vi "_FPGA System Polling.vi"(4 "error in (no error)":errorcluster, 5 "Waiting (F)":bool, 6 "Connected?":bool, 7 "CurInstrState":T3) -> (1 "Running":bool, 3 "Next InstrState":T3)   [LabVIEW 2012]
uses:
  Type/_RT Instrument State.ctl
  Type/_RT Polling Settings.ctl
  Type/_LCD Line2 Msg.ctl
  Type/_LED States.ctl
  Type/_LCD Line1 Msg.ctl
  Type/_RW Status.ctl
  Type/_Pump Parameter.ctl
  _RT Global.vi
  <vilib>/Utility/error.llb/Error Cluster From Error Code.vi
  <vilib>/rvi/errors/niLvFpgaAdjustHostInterfaceError.vi
  <vilib>/rvi/interface/nirviReadWriteControl/nirviReadWriteControl.xnode
  FPGA Bitfiles/FPGA9606.lvbitx
  NiFpgaLv.dll
panel:
  in  "Polling Settings":T1[](array[typedef])=[{"ADC Ch"=119, "UserVal"=FALSE, "LowVal"=0.0, "HighVal"=89.0, "Fail Level"=50, "Err"="VG Disconnected/Broken Warning", "Line2Msg"=13, "InstrState"=enum."Ready", "Code"="004"}, {"ADC Ch"=119, "UserVal"=FALSE, "LowVal"=255.0, "HighVal"=300.0, "Fail Level"=50, "Err"="VG Disconnected/Broken Warning", "Line2Msg"=13, "InstrState"=enum."Ready", "Code"="004"}, {"ADC Ch"=119, "UserVal"=FALSE, "LowVal"=150.0, "HighVal"=254.0, "Fail Level"=50, "Err"="Overpressure Warning", "Line2Msg"=13, "InstrState"=enum."Ready", "Code"="006"}, {"ADC Ch"=64, "UserVal"=FALSE, "LowVal"=-5.0, "HighVal"=0.249, "Fail Level"=39, "Err"="Drying Gas Low", "Line2Msg"=4, "InstrState"=enum."Turbopump Ready", "Code"=""}, {"ADC Ch"=74, "UserVal"=FALSE, "LowVal"=0.36, "HighVal"=5.0, "Fail Level"=10, "Err"="Foreline Pressure Failure", "Line2Msg"=2, "InstrState"=enum."Fault", "Code"="001"}, {"ADC Ch"=25, "UserVal"=TRUE, "LowVal"=91.0, "HighVal"=200.0, "Fail Level"=35, "Err"="Q2 Board Slot 5 Overheating", "Line2Msg"=5, "InstrState"=enum."Turbopump Ready-Waiting", "Code"="008"}, {"ADC Ch"=49, "UserVal"=TRUE, "LowVal"=91.0, "HighVal"=200.0, "Fail Level"=35, "Err"="Q1 Board Slot 9 Overheating", "Line2Msg"=5, "InstrState"=enum."Turbopump Ready-Waiting", "Code"="009"}, {"ADC Ch"=57, "UserVal"=TRUE, "LowVal"=91.0, "HighVal"=200.0, "Fail Level"=35, "Err"="M1RF Board Slot 13 Overheating", "Line2Msg"=5, "InstrState"=enum."Turbopump Ready-Waiting", "Code"="010"}, {"ADC Ch"=26, "UserVal"=TRUE, "LowVal"=91.0, "HighVal"=200.0, "Fail Level"=35, "Err"="Q2 Board Slot 5 Overheating", "Line2Msg"=5, "InstrState"=enum."Turbopump Ready-Waiting", "Code"="008"}, {"ADC Ch"=50, "UserVal"=TRUE, "LowVal"=91.0, "HighVal"=200.0, "Fail Level"=35, "Err"="Q1 Board Slot 9 Overheating", "Line2Msg"=5, "InstrState"=enum."Turbopump Ready-Waiting", "Code"="009"}, {"ADC Ch"=58, "UserVal"=TRUE, "LowVal"=91.0, "HighVal"=200.0, "Fail Level"=35, "Err"="M1RF Board Slot 13 Overheating", "Line2Msg"=5, "InstrState"=enum."Turbopump Ready-Waiting", "Code"="010"}, {"ADC Ch"=113, "UserVal"=FALSE, "LowVal"=1.0, "HighVal"=2.0, "Fail Level"=40, "Err"="Source 1 Interlock Activated", "Line2Msg"=6, "InstrState"=enum."Source Standby", "Code"=""}, {"ADC Ch"=114, "UserVal"=FALSE, "LowVal"=1.0, "HighVal"=2.0, "Fail Level"=40, "Err"="Source 2 Interlock Activated", "Line2Msg"=7, "InstrState"=enum."Source Standby", "Code"=""}, {"ADC Ch"=14, "UserVal"=FALSE, "LowVal"=4.5, "HighVal"=10.0, "Fail Level"=35, "Err"="Heater PS Current High", "Line2Msg"=8, "InstrState"=enum."Turbopump Ready-Waiting", "Code"="011"}, {"ADC Ch"=51, "UserVal"=TRUE, "LowVal"=-9999.0, "HighVal"=-12.0, "Fail Level"=35, "Err"="Q1 Tuning Error", "Line2Msg"=5, "InstrState"=enum."Turbopump Ready-Waiting", "Code"="012"}, {"ADC Ch"=27, "UserVal"=TRUE, "LowVal"=-9999.0, "HighVal"=-12.0, "Fail Level"=35, "Err"="Q2 Tuning Error", "Line2Msg"=5, "InstrState"=enum."Turbopump Ready-Waiting", "Code"="013"}, {"ADC Ch"=59, "UserVal"=TRUE, "LowVal"=-9999.0, "HighVal"=-12.0, "Fail Level"=35, "Err"="M1 Tuning Error", "Line2Msg"=5, "InstrState"=enum."Turbopump Ready-Waiting", "Code"="014"}, {"ADC Ch"=120, "UserVal"=FALSE, "LowVal"=0.0, "HighVal"=0.0, "Fail Level"=32, "Err"="Card Cage Door Interlock Activated", "Line2Msg"=9, "InstrState"=enum."Go to 24V Standby", "Code"=""}, {"ADC Ch"=121, "UserVal"=FALSE, "LowVal"=0.0, "HighVal"=0.0, "Fail Level"=35, "Err"="Vacuum Ready Tripped", "Line2Msg"=2, "InstrState"=enum."Turbopump Ready-Waiting", "Code"="015"}, {"ADC Ch"=76, "UserVal"=FALSE, "LowVal"=0.0, "HighVal"=2.5, "Fail Level"=39, "Err"="Drying Gas Supply Low", "Line2Msg"=4, "InstrState"=enum."Turbopump Ready", "Code"=""}, {"ADC Ch"=78, "UserVal"=FALSE, "LowVal"=0.0, "HighVal"=3.5, "Fail Level"=39, "Err"="Source Gas Supply Low", "Line2Msg"=12, "InstrState"=enum."Turbopump Ready", "Code"=""}, {"ADC Ch"=100, "UserVal"=FALSE, "LowVal"=0.0, "HighVal"=0.0, "Fail Level"=32, "Err"="Electronics is off", "Line2Msg"=5, "InstrState"=enum."Go to 24V Standby", "Code"="017"}, {"ADC Ch"=72, "UserVal"=FALSE, "LowVal"=4.6, "HighVal"=5.1, "Fail Level"=50, "Err"="Exhaust Gas Low", "Line2Msg"=0, "InstrState"=enum."Ready", "Code"=""}, {"ADC Ch"=81, "UserVal"=TRUE, "LowVal"=26.0, "HighVal"=30.0, "Fail Level"=50, "Err"="RF Board Power Supply Error", "Line2Msg"=0, "InstrState"=enum."Ready", "Code"=""}, {"ADC Ch"=82, "UserVal"=TRUE, "LowVal"=-30.0, "HighVal"=-26.0, "Fail Level"=50, "Err"="RF Board Power Supply Error", "Line2Msg"=0, "InstrState"=enum."Ready", "Code"=""}, {"ADC Ch"=83, "UserVal"=TRUE, "LowVal"=56.0, "HighVal"=62.0, "Fail Level"=50, "Err"="Heater Power Supply Error", "Line2Msg"=0, "InstrState"=enum."Ready", "Code"=""}, {"ADC Ch"=85, "UserVal"=TRUE, "LowVal"=22.0, "HighVal"=26.0, "Fail Level"=50, "Err"="24 V Mains Power Supply Error", "Line2Msg"=0, "InstrState"=enum."Ready", "Code"=""}, {"ADC Ch"=86, "UserVal"=TRUE, "LowVal"=13.0, "HighVal"=16.0, "Fail Level"=50, "Err"="ADC/Board Power Supply Error", "Line2Msg"=0, "InstrState"=enum."Ready", "Code"=""}, {"ADC Ch"=87, "UserVal"=TRUE, "LowVal"=-16.0, "HighVal"=-13.0, "Fail Level"=50, "Err"="ADC/Board Power Supply Error", "Line2Msg"=0, "InstrState"=enum."Ready", "Code"=""}] {"Line2Msg" items=["Same", "Empty", "VacFail", "Cancel", "CheckGas", "EleFail", "Probe1Fail", "Probe2Fail", "HeaterFail", "DoorOpen", "CheckComm", "PressStart", "CheckSource", "VacWarn", "ForelineHigh"]}
  # "0   119  50 vacuum gauge disconnected\n1   119  50 vacuum gauge disconnected\n2   119  50 overpressure warning\n3   64    39 drying gas low\n4   74    10 foreline pressure failure\n5   25    35 Q2 board slot 5 overheating\n6   49    35 Q1 board slot 9 overheating\n7   57    35 M1RF board slot 13 overheating\n8   26    35 Q2 board slot 5 overheating\n9   50    35 Q1 board slot 9 overheating\n10  58    35 M1RF board slot 13 overheating\n11 113  40 source 1 interlock activated\n12 114  40 source 2 interlock activated\n13  14    35 heater PS currect high\n14  51    35 Q1 tuning error\n15  27    35 Q2 tuning error\n16  59    35 M1 tuning error\n17 120  32 card cage door interlock activated\n18 121  35 vacuum ready tripped\n19  76    40 drying gas supply low\n20  78    40 source gas supply low\n21 100  32 electronics is off\n22  72    50 exhaust gas low\n23  81    50 RF board power supply error\n24  82    50 RF board power supply error\n25  83    50 heater power supply error\n26  85    50 24 V mains power supply error\n27  86    50 ADC/board power supply error\n28  87    50 ADC/board power supply error"
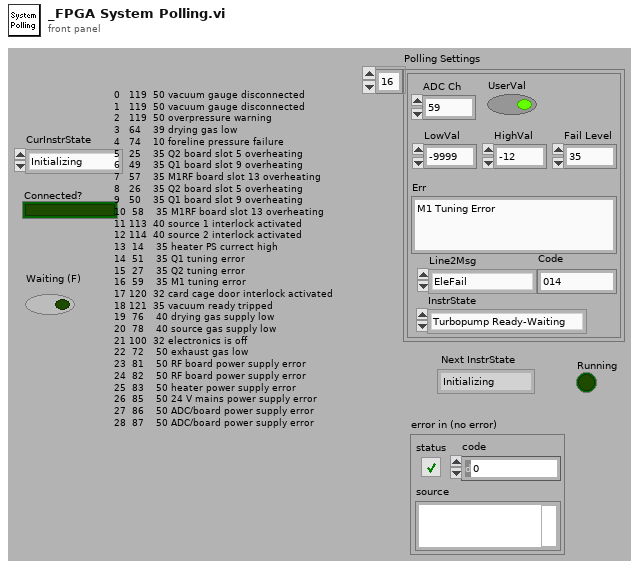
[diagram p1: front panel]
types:
  T1 = typedef "_RT Polling Settings.ctl" = cluster{"ADC Ch":u8, "UserVal":bool, "LowVal":sgl, "HighVal":sgl, "Fail Level":u8, "Err":string, "Line2Msg":T2, "InstrState":T3, "Code":string}
  T2 = typedef "_LCD Line2 Msg.ctl" = u16
  T3 = typedef "_RT Instrument State.ctl" = enum16{"Initializing", "Mass Spectrometer is Off", "Starting Up", "Turning Power Off", "Going to Standby", "Roughing Pump Ready", "Turning Turbo Off", "Turbo Startup", "Turbopump Ready", "Checking Vacuum", "Going to Ready", "Ready", "Running", "Source Standby", "Lost Communication", "Shutting Down", "Fault", "24V Standby", "Go to 24V Standby", "Turbopump Ready-Waiting"}
  T4 = typedef "_RT Startup Options.ctl" = cluster{"Door":bool, "Curtain":bool, "Pressure":bool, "Turbo":bool, "SysPoll":bool, "GasFlag":bool}
  T5 = typedef "_LED States.ctl" = enum8{"Idle", "Solid B", "Solid R", "Solid P", "Off B", "Off R", "Off P", "Off BRP", "Off RP", "Flash R&P", "Flash P"}
  T6 = typedef "_Pump Parameter.ctl" = enum16{"Turn Pump Motor On", "Turn Pump Motor Off", "Read Pump Oil Deficiency", "Read Rotation Switch Point Attained", "Read Ele. Drive Over Temperature", "Read Pump Over Temperature", "Read Set Rotation Speed Attained", "Read Turbopump Accelerates", "Read Actual Rotation Speed in Hz", "Read Motor Current in A", "Read Operating Hours in h", "Read Motor Voltage in V", "Read Motor Power in W", "Set Rotation Speed Switchpoint in %", "Clear Error", "Read Error Code", "Read Bearing Temperature", "Read Hardware Version", "Read Firmware Version", "Read Operating Hours (Drive)", "Read Rotational Speed (rpm)", "Read Power Stage Temperature", "Read Electronics Temperature", "Read Upper Pump Temperature", "Read Motor Temperature", "Read Error Code History, 1", "Read Error Code History, 2", "Read Error Code History, 3", "Read Error Code History, 4", "Read Error Code History, 5", "Read Error Code History, 6", "Read Error Code History, 7", "Read Error Code History, 8", "Read Error Code History, 9", "Read Error Code History, 10"}
  T7 = typedef "_RW Status.ctl" = enum8{"Done", "Do Read", "Do Write", "Set Latch1", "Set Latch2", "Set Latch3", "Set Latch4", "RP ON", "EL ON", "Serial Send", "Set LC Out", "Get LC In", "Read VAC", "Table Test", "Get Interlock", "Do Read2", "Do Write2"}
  T8 = typedef "_LCD Line1 Msg.ctl" = u16
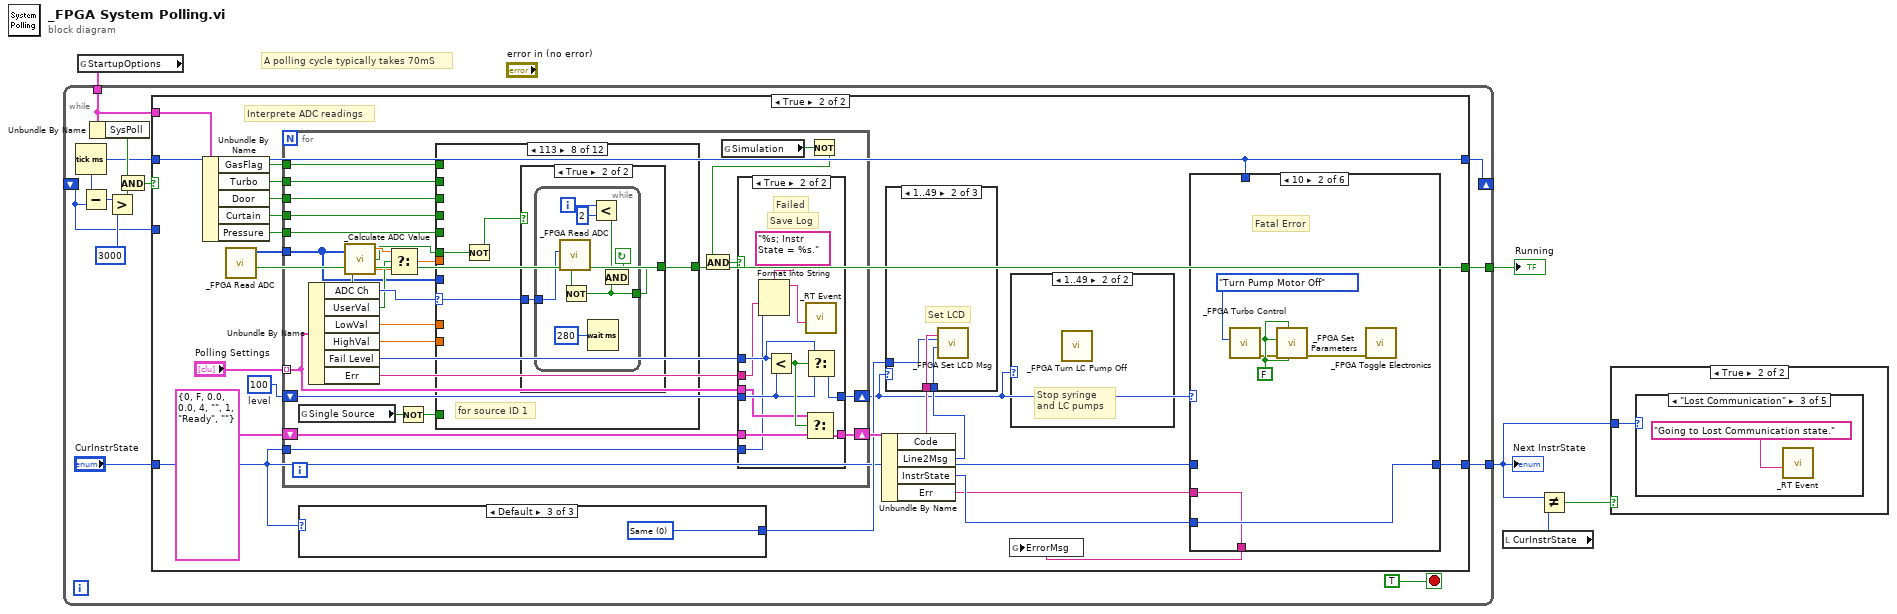
[diagram p0: block diagram]
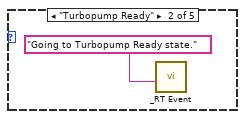
[diagram p4: hidden frame]
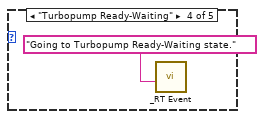
[diagram p5: hidden frame]
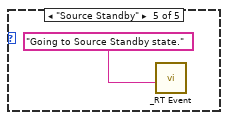
[diagram p6: hidden frame]
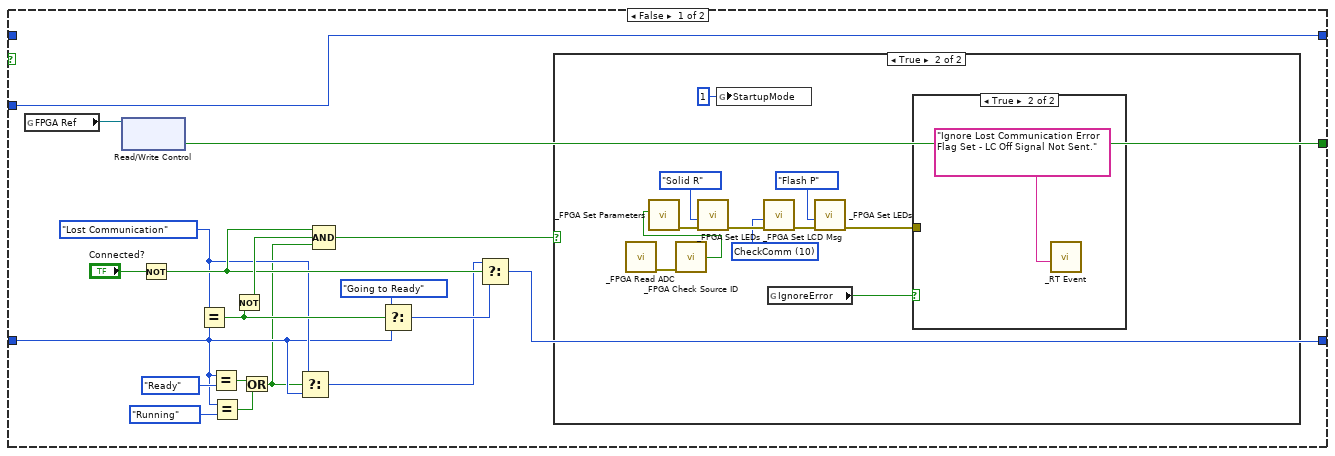
[diagram p7: hidden frame]
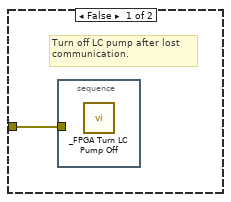
[diagram p9: hidden frame]
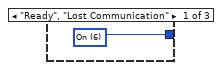
[diagram p11: hidden frame]
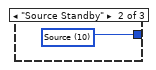
[diagram p12: hidden frame]
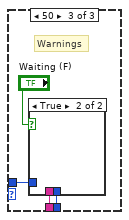
[diagram p14: hidden frame]
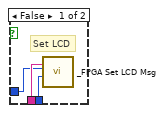
[diagram p15: hidden frame]
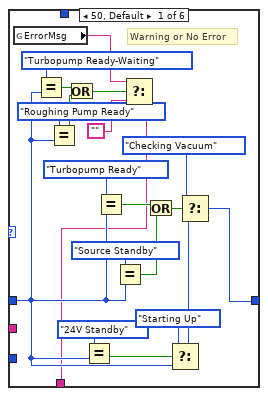
[diagram p16: hidden frame]
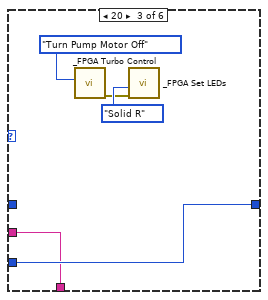
[diagram p17: hidden frame]
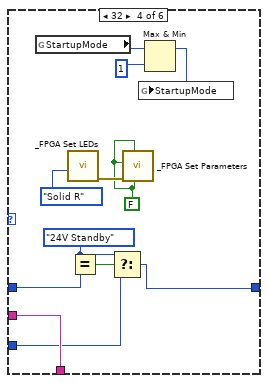
[diagram p18: hidden frame]
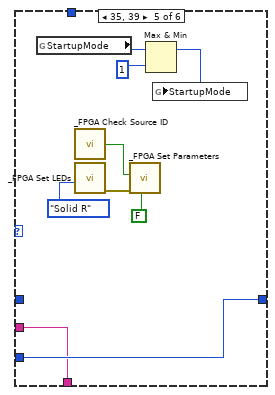
[diagram p19: hidden frame]
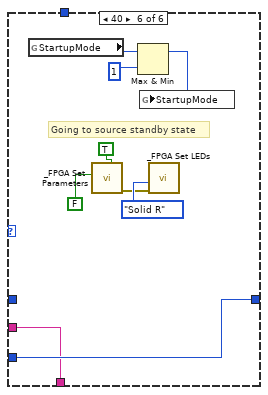
[diagram p20: hidden frame]
diagram:
  # "A polling cycle typically takes 70mS"
  n1 = global read "_RT Global.vi" "StartupOptions"() -> (w4:T4)
  n2 = while {
    tunnel: [w16] -> w1
    shift-right: [w7] -> _
    shift-left: _ -> [w6]
    tunnel: [w13] -> w5
    tunnel: w4 -> [w9]
    stop <- TRUE stop-if-true
    n3 = Tick Count (ms)() -> (millisecond timer value=w8:u32)
    n4 = Subtract(x=w8, y=w6) -> (x-y=w15:u32)
    n5 = Unbundle By Name(w9) -> ("SysPoll"=w12:bool)
    n6 = Greater?(x=w15, y=3000) -> (0:w11:bool)
    n7 = And(x=w12, y=w11) -> (x .and. y?=w10:bool)
    n8 = case shown="True" w10 {
      tunnel: [w30 w69] -> w16
      tunnel: "CurInstrState" -> [w22 w52]
      tunnel: [w28 w72] -> w13
      tunnel: w9 -> [_ w67]
      tunnel: w8 -> [_ w51]
      tunnel: [w32 w51] -> w7
      tunnel: w6 -> [w32 _]
      frame False {
        w23 = _RT_Instrument_State."Lost Communication" ("t")
        n9 = global read "_RT Global.vi" "FPGA Ref"() -> (w19:refnum<k20>)
        n10 = xnode "Read/Write Control"("FPGA VI Reference In"=w19) -> ("Running"=w28:bool)  [unwired: 1 in, 2 out]
        n11 = Not(x="Connected?") -> (.not. x?=w31:bool)
        n12 = Equal?(x=w23, y=w22) -> (x = y?=w35:bool)
        n13 = Equal?(x=w22, y=_RT_Instrument_State."Ready") -> (x = y?=w25:bool)
        n14 = Equal?(x=w22, y=_RT_Instrument_State."Running") -> (x = y?=w24:bool)
        n15 = Not(x=w35) -> (.not. x?=w34:bool)
        n16 = Or(x=w25, y=w24) -> (x .or. y?=w20:bool)
        n17 = Select(t=w23, s=w20, f=w22) -> (s? t:f=w21:T3)
        n18 = Compound Arithmetic op=AND(w31, w34, w20) -> (w33:bool)
        n19 = Select(t=_RT_Instrument_State."Going to Ready", s=w35, f=w22) -> (s? t:f=w36:T3)
        n20 = Select(t=w21, s=w31, f=w36) -> (s? t:f=w30:T3)
        n21 = case shown="True" w33 {
          frame False {
          }
          frame True {
            w42 = T2 10 items=["Same", "Empty", "VacFail", "Cancel", "CheckGas", "EleFail", "Probe1Fail", "Probe2Fail", "HeaterFail", "DoorOpen", "CheckComm", "PressStart", "StartRP"] ("Line2Msg (same)")
            n22 = call "_FPGA Read ADC.vi"() -> ("error out"=w44:errorcluster)  [unwired: 3 in, 6 out]
            n23 = call "_FPGA Check Source ID.vi"("error in (no error)"=w44) -> ("Source ID OK"=w43:bool)
            n24 = call "_FPGA Set Parameters.vi"("HSID Temp (on)"=w43) -> ("error out"=w40:errorcluster)  [unwired: 8 in, 2 out]
            n25 = call "_FPGA Set LEDs.vi"("error in (no error)"=w40, "LED Command"=_LED_States."Solid R") -> ("error out"=w47:errorcluster)  [unwired: 2 in, 3 out]
            n26 = global write "_RT Global.vi" "StartupMode"(u8 1 ("StartupMode")) -> ()
            n27 = call "_FPGA Set LCD Msg.vi"("error in"=w47, "Line2Msg (same)"=w42) -> ("error out"=w45:errorcluster)  [unwired: 5 in, 2 out]
            n28 = global read "_RT Global.vi" "IgnoreError"() -> (w38:bool)
            n29 = call "_FPGA Set LEDs.vi"("error in (no error)"=w45, "LED Command"=_LED_States."Flash P") -> ("error out"=w39:errorcluster)  [unwired: 2 in, 3 out]
            n30 = case shown="True" w38 {
              tunnel: w39 -> [w49 _]
              frame False {
                # "Turn off LC pump after lost\ncommunication."
                n31 = stacked-sequence {
                  tunnel: w49 -> [_]
                  frame #0 {
                    n32 = call "_FPGA Turn LC Pump Off.vi"() -> ()  [unwired: 2 in]
                  }
                }
              }
              frame True {
                n33 = call "_RT Event.vi"("Event"="Ignore Lost Communication Error Flag Set - LC Off Signal Not Sent.") -> ()  [unwired: 2 in, 5 out]
              }
            }
          }
        }
      }
      frame True {
        w70 = u8 100  # level
        # "Interprete ADC readings"
        n34 = Unbundle By Name(w67) -> ("GasFlag"=w56:bool, "Turbo"=w63:bool, "Door"=w66:bool, "Curtain"=w65:bool, "Pressure"=w64:bool)
        n35 = call "_FPGA Read ADC.vi"() -> ("Running"=w72:bool, "ADC Values"=w71:i32[])  [unwired: 3 in, 5 out]
        n36 = for {
          tunnel: w71 -> [w149]
          shift-right: [w166] -> w55
          shift-left: w70 -> [w168]
          tunnel: "Polling Settings" -> [w156] mode=indexing
          shift-right: [w165] -> w61
          shift-left: T1 {"ADC Ch"=0, "UserVal"=FALSE, "LowVal"=0.0, "HighVal"=0.0, "Fail Level"=4, "Err"="", "Line2Msg"=1, "InstrState"=enum."Ready", "Code"=""} ("Cluster") -> [w167]
          tunnel: w66 -> [w160]
          tunnel: w65 -> [w159]
          tunnel: w64 -> [w158]
          tunnel: w63 -> [w157]
          tunnel: w56 -> [w155]
          tunnel: w52 -> [w147]
          n37 = global read "_RT Global.vi" "Single Source"() -> (w154:bool)
          n38 = Unbundle By Name(w156) -> ("ADC Ch"=w174:u8, "UserVal"=w173:bool, "LowVal"=w170:sgl, "HighVal"=w169:sgl, "Fail Level"=w164:u8, "Err"=w163:string)
          n39 = call "_Calculate ADC Value.vi"("ADC Values"=w149, "ADC Channel (64)"=w174) -> ("User Value"=w172:sgl, "In Range?"=w148:bool, "Raw Reading"=w171:sgl)
          n40 = Select(t=w172, s=w173, f=w171) -> (s? t:f=w161:sgl)
          n41 = Not(x=w154) -> (.not. x?=w153:bool)
          n42 = case shown="113" w174 {
            selector: w174 -> [_ _ _ w200 _ w234 _ w272 w288 _ _ _]
            tunnel: w161 -> [w191 w196 _ w206 w230 _ w257 _ _ _ _ _]
            tunnel: w170 -> [w190 w195 _ w202 w229 _ w252 _ _ _ _ _]
            tunnel: w169 -> [w189 w194 _ w203 w228 _ w251 _ _ _ _ _]
            tunnel: [w188 w192 FALSE w201 w226 w235 w253 w273 w290 w309 FALSE w346] -> w162
            tunnel: w160 -> [_ _ _ _ _ _ _ _ _ w311 _ _]
            tunnel: w159 -> [_ _ _ w199 _ _ _ _ _ _ _ _]
            tunnel: w158 -> [_ _ _ _ w225 _ _ _ _ _ _ _]
            tunnel: w157 -> [_ _ _ _ _ _ w255 _ _ _ _ _]
            tunnel: w155 -> [_ _ _ _ _ w233 _ _ _ _ _ _]
            tunnel: w153 -> [_ _ _ _ _ _ _ _ w287 _ _ _]
            tunnel: w149 -> [_ _ _ _ _ _ _ _ _ _ w339 _]
            tunnel: w148 -> [_ _ w197 _ _ w232 _ w275 w291 w308 _ w347]
            frame Default {
              # "Range in Error"
              n43 = In Range and Coerce(upper limit=w189, x=w191, lower limit=w190) -> (In Range?=w188:bool)  [unwired: 1 out]
            }
            frame 20..23, 81..97 {
              # "Allowable Range"
              n44 = In Range and Coerce(upper limit=w194, x=w196, lower limit=w195) -> (In Range?=w193:bool)  [unwired: 1 out]
              n45 = Not(x=w193) -> (.not. x?=w192:bool)
            }
            frame 72 {
              # "Check for exhaust gas"
              n46 = Not(x=w197) -> ()  [unwired: 1 out]
            }
            frame 64 {
              # "Curtain Gas"
              n47 = In Range and Coerce(upper limit=w203, x=w206, lower limit=w202) -> (In Range?=w205:bool)  [unwired: 1 out]
              n48 = And(x=w199, y=w205) -> (x .and. y?=w204:bool)
              n49 = case shown="True" w204 {
                selector: w204 -> [w207 _]
                tunnel: [w207 w212] -> w201
                tunnel: w202 -> [_ w211]
                tunnel: w203 -> [_ w210]
                tunnel: w200 -> [_ w209]
                tunnel: w199 -> [_ w208]
                frame False {
                }
                frame True {
                  n50 = while {
                    tunnel: [w213] -> w212
                    tunnel: w211 -> [w224]
                    tunnel: w210 -> [w223]
                    tunnel: w209 -> [w217]
                    tunnel: w208 -> [w216]
                    i -> [w222]
                    stop <- w220 continue-if-true
                    n51 = call "_FPGA Read ADC.vi"("ADC Channel (64)"=w217) -> ("Raw Reading"=w218:sgl)  [unwired: 2 in, 6 out]
                    n52 = In Range and Coerce(upper limit=w223, x=w218, lower limit=w224) -> (In Range?=w215:bool)  [unwired: 1 out]
                    n53 = Less?(x=w222, y=2) -> (x < y?=w214:bool)
                    n54 = Wait (ms)(milliseconds to wait=u32 280) -> ()  [unwired: 1 out]
                    n55 = And(x=w216, y=w215) -> (x .and. y?=w213:bool)
                    n56 = And(x=w213, y=w214) -> (x .and. y?=w220:bool)
                  }
                }
              }
            }
            frame 74 {
              # "Foreline Pressure"
              n57 = In Range and Coerce(upper limit=w228, x=w230, lower limit=w229) -> (In Range?=w227:bool)  [unwired: 1 out]
              n58 = And(x=w225, y=w227) -> (x .and. y?=w226:bool)
            }
            frame 76, 78 {
              # "For Auto Gas Flags"
              n59 = Not(x=w232) -> (.not. x?=w231:bool)
              n60 = And(x=w233, y=w231) -> (x .and. y?=w236:bool)
              n61 = case shown="True" w236 {
                selector: w236 -> [w237 _]
                tunnel: [w237 w240] -> w235
                tunnel: w234 -> [_ w239]
                tunnel: w233 -> [_ w238]
                frame False {
                }
                frame True {
                  n62 = while {
                    tunnel: [w243] -> w240
                    tunnel: w239 -> [w246]
                    tunnel: w238 -> [w245]
                    i -> [w250]
                    stop <- w248 continue-if-true
                    n63 = call "_FPGA Read ADC.vi"("ADC Channel (64)"=w246) -> ("In Range?"=w242:bool)  [unwired: 2 in, 6 out]
                    n64 = Not(x=w242) -> (.not. x?=w241:bool)
                    n65 = Less?(x=w250, y=2) -> (x < y?=w244:bool)
                    n66 = Wait (ms)(milliseconds to wait=u32 280) -> ()  [unwired: 1 out]
                    n67 = And(x=w245, y=w241) -> (x .and. y?=w243:bool)
                    n68 = And(x=w243, y=w244) -> (x .and. y?=w248:bool)
                  }
                }
              }
            }
            frame 119 {
              # "High Pressure"
              n69 = In Range and Coerce(upper limit=w251, x=w257, lower limit=w252) -> (In Range?=w256:bool)  [unwired: 1 out]
              n70 = And(x=w255, y=w256) -> (x .and. y?=w254:bool)
              n71 = case shown="True" w254 {
                selector: w254 -> [w258 _]
                tunnel: [w258 w261] -> w253
                tunnel: w252 -> [_ w260]
                tunnel: w251 -> [_ w259]
                frame False {
                }
                frame True {
                  n72 = while {
                    tunnel: [w265] -> w261
                    tunnel: w260 -> [w271]
                    tunnel: w259 -> [w270]
                    i -> [w267]
                    stop <- w263 continue-if-true
                    n73 = call "_FPGA Read Data.vi"("Read Mode (Do Read)"=_RW_Status."Read VAC" ("R/W Status")) -> ("Data"=w268:u32)  [unwired: 4 in, 2 out]
                    n74 = In Range and Coerce(upper limit=w270, x=w268, lower limit=w271) -> (In Range?=w265:bool)  [unwired: 1 out]
                    n75 = Less?(x=w267, y=4) -> (x < y?=w264:bool)
                    n76 = Wait (ms)(milliseconds to wait=u32 180) -> ()  [unwired: 1 out]
                    n77 = And(x=w264, y=w265) -> (x .and. y?=w263:bool)
                  }
                }
              }
            }
            frame 113 {
              # "for source ID 1"
              n78 = Not(x=w275) -> (.not. x?=w274:bool)
              n79 = case shown="True" w274 {
                selector: w274 -> [w276 _]
                tunnel: [w276 w278] -> w273
                tunnel: w272 -> [_ w277]
                frame False {
                }
                frame True {
                  n80 = while {
                    tunnel: [w279] -> w278
                    tunnel: w277 -> [w281]
                    i -> [w286]
                    stop <- w283 continue-if-true
                    n81 = call "_FPGA Read ADC.vi"("ADC Channel (64)"=w281) -> ("In Range?"=w280:bool)  [unwired: 2 in, 6 out]
                    n82 = Not(x=w280) -> (.not. x?=w279:bool)
                    n83 = Wait (ms)(milliseconds to wait=u32 280) -> ()  [unwired: 1 out]
                    n84 = Less?(x=w286, y=2) -> (x < y?=w284:bool)
                    n85 = And(x=w284, y=w279) -> (x .and. y?=w283:bool)
                  }
                }
              }
            }
            frame 114 {
              # "for source ID 2"
              n86 = Not(x=w291) -> (.not. x?=w292:bool)
              n87 = And(x=w292, y=w287) -> (x .and. y?=w289:bool)
              n88 = case shown="True" w289 {
                selector: w289 -> [w293 _]
                tunnel: [w293 w296] -> w290
                tunnel: w288 -> [_ w295]
                tunnel: w287 -> [_ w294]
                frame False {
                }
                frame True {
                  n89 = while {
                    tunnel: [w297] -> w296
                    tunnel: w295 -> [w301]
                    tunnel: w294 -> [w299]
                    i -> [w306]
                    stop <- w303 continue-if-true
                    n90 = call "_FPGA Read ADC.vi"("ADC Channel (64)"=w301) -> ("In Range?"=w300:bool)  [unwired: 2 in, 6 out]
                    n91 = Not(x=w300) -> (.not. x?=w298:bool)
                    n92 = Wait (ms)(milliseconds to wait=u32 280) -> ()  [unwired: 1 out]
                    n93 = And(x=w298, y=w299) -> (x .and. y?=w297:bool)
                    n94 = Less?(x=w306, y=2) -> (x < y?=w304:bool)
                    n95 = And(x=w304, y=w297) -> (x .and. y?=w303:bool)
                  }
                }
              }
            }
            frame 120 {
              # "for door interlock"
              n96 = Not(x=w308) -> (.not. x?=w307:bool)
              n97 = And(x=w311, y=w307) -> (x .and. y?=w310:bool)
              n98 = case shown="True" w310 {
                selector: w310 -> [w312 _]
                tunnel: [w312 w313] -> w309
                frame False {
                }
                frame True {
                  # "if fail, do a direct read"
                  n99 = call "_FPGA Read Data.vi"("Read Mode (Do Read)"=_RW_Status."Get Interlock" ("R/W Status")) -> ("Data"=w314:u32)  [unwired: 4 in, 2 out]
                  n100 = Equal To 0?(x=w314) -> (x = 0?=w313:bool)
                }
              }
            }
            frame 100 {
              w317 = sgl 0.5 ("y")
              # "Check for electronics off"
              n101 = global read "_RT Global.vi" "Ele On"() -> (w325:bool)
              n102 = call "_Calculate ADC Value.vi"("ADC Values"=w339, "ADC Channel (64)"=u8 20) -> ("Raw Reading"=w338:sgl)  [unwired: 2 out]
              n103 = call "_Calculate ADC Value.vi"("ADC Values"=w339, "ADC Channel (64)"=u8 21) -> ("Raw Reading"=w336:sgl)  [unwired: 2 out]
              n104 = call "_Calculate ADC Value.vi"("ADC Values"=w339, "ADC Channel (64)"=u8 88) -> ("Raw Reading"=w335:sgl)  [unwired: 2 out]
              n105 = call "_Calculate ADC Value.vi"("ADC Values"=w339, "ADC Channel (64)"=u8 89) -> ("Raw Reading"=w334:sgl)  [unwired: 2 out]
              n106 = call "_Calculate ADC Value.vi"("ADC Values"=w339, "ADC Channel (64)"=u8 96) -> ("Raw Reading"=w333:sgl)  [unwired: 2 out]
              n107 = call "_Calculate ADC Value.vi"("ADC Values"=w339, "ADC Channel (64)"=u8 97) -> ("Raw Reading"=w337:sgl)  [unwired: 2 out]
              n108 = Absolute Value(x=w337) -> (abs(x)=w318:sgl)
              n109 = Absolute Value(x=w336) -> (abs(x)=w322:sgl)
              n110 = Absolute Value(x=w333) -> (abs(x)=w319:sgl)
              n111 = Absolute Value(x=w338) -> (abs(x)=w323:sgl)
              n112 = Absolute Value(x=w334) -> (abs(x)=w320:sgl)
              n113 = Absolute Value(x=w335) -> (abs(x)=w321:sgl)
              n114 = Not(x=w325) -> (.not. x?=w326:bool)
              n115 = Less?(x=w323, y=w317) -> (x < y?=w332:bool)
              n116 = Less?(x=w322, y=w317) -> (x < y?=w329:bool)
              n117 = Less?(x=w321, y=w317) -> (x < y?=w330:bool)
              n118 = Less?(x=w320, y=w317) -> (x < y?=w328:bool)
              n119 = Less?(x=w319, y=w317) -> (x < y?=w327:bool)
              n120 = Less?(x=w318, y=w317) -> (x < y?=w331:bool)
              n121 = Compound Arithmetic op=AND(w332, w329, w330, w328, w327, w331) -> (w324:bool)
              n122 = Or(x=w326, y=w324) -> ()  [unwired: 1 out]
            }
            frame 121 {
              # "for vacuum ready interlock"
              n123 = Not(x=w347) -> (.not. x?=w346:bool)
            }
          }
          n124 = global read "_RT Global.vi" "Simulation"() -> (w152:bool)
          n125 = Not(x=w152) -> (.not. x?=w150:bool)
          n126 = And(x=w150, y=w162) -> (x .and. y?=w151:bool)
          n127 = case shown="True" w151 {
            tunnel: w168 -> [w176 w185]
            tunnel: [w176 w184] -> w166
            tunnel: w164 -> [_ w186]
            tunnel: w167 -> [w175 w181]
            tunnel: [w175 w183] -> w165
            tunnel: w163 -> [_ w179]
            tunnel: w156 -> [_ w182]
            tunnel: w147 -> [_ w178]
            frame False {
              # "Passed"
            }
            frame True {
              # "Save Log"
              # "Failed"
              n128 = Format Into String(format string="%s; Instr State = %s.", w179, w178) -> (resulting string=w177:string)  [unwired: 2 in, 1 out]
              n129 = Less?(x=w186, y=w185) -> (x < y?=w187:bool)
              n130 = Select(t=w182, s=w187, f=w181) -> (s? t:f=w183:T1)
              n131 = call "_RT Event.vi"("Event"=w177) -> ()  [unwired: 2 in, 5 out]
              n132 = Select(t=w186, s=w187, f=w185) -> (s? t:f=w184:u8)
            }
          }
        }
        n133 = case shown="Default" w52 {
          tunnel: [w73 w74 w75] -> w57
          frame "Ready", "Lost Communication" {
            w73 = T8 6 items=["Same", "Empty", "Connected", "Starting", "Stopping", "Action", "On", "Service", "Call", "Acquiring", "Source"] ("Line1Msg (same)")
          }
          frame "Source Standby" {
            w74 = T8 10 items=["Same", "Empty", "Connected", "Starting", "Stopping", "Action", "On", "Service", "Call", "Acquiring", "Source"] ("Line1Msg (same)")
          }
          frame Default {
            w75 = T8 0 items=["Same", "Empty", "Connected", "Starting", "Stopping", "Action", "On", "Service", "Call", "Acquiring", "Source"] ("Line1Msg (same)")
          }
        }
        n134 = Unbundle By Name(w61) -> ("Code"=w58:string, "Line2Msg"=w59:T2, "InstrState"=w60:T3, "Err"=w54:string)
        n135 = case shown="1..49" w55 {
          tunnel: w59 -> [_ w78 w82]
          tunnel: w58 -> [_ w77 w81]
          tunnel: w57 -> [_ w76 w80]
          frame Default {
          }
          frame 1..49 {
            # "Set LCD"
            n136 = call "_FPGA Set LCD Msg.vi"("ErrNum"=w77, "Line2Msg (same)"=w78, "Line1Msg (same)"=w76) -> ()  [unwired: 4 in, 3 out]
          }
          frame 50 {
            # "Warnings"
            n137 = case shown="True" "Waiting (F)" {
              tunnel: w82 -> [w85 _]
              tunnel: w81 -> [w84 _]
              tunnel: w80 -> [w83 _]
              frame False {
                # "Set LCD"
                n138 = call "_FPGA Set LCD Msg.vi"("ErrNum"=w84, "Line2Msg (same)"=w85, "Line1Msg (same)"=w83) -> ()  [unwired: 4 in, 3 out]
              }
              frame True {
              }
            }
          }
        }
        n139 = case shown="1..49" w55 {
          frame 0, Default {
          }
          frame 1..49 {
            # "Stop syringe \nand LC pumps"
            n140 = call "_FPGA Turn LC Pump Off.vi"() -> ()  [unwired: 2 in]
          }
        }
        n141 = case shown="10" w55 {
          tunnel: w52 -> [w92 _ _ w124 _ _]
          tunnel: [w99 w109 w114 w120 w133 w144] -> w69
          tunnel: w60 -> [_ w109 w114 w121 w133 w144]
          tunnel: w54 -> [_ w108 w113 w125 w132 w142]
          tunnel: [w86 w108 w113 w125 w132 w142] -> w53
          tunnel: w51 -> [_ _ _ _ _ _]
          frame 50, Default {
            # "Warning or No Error"
            n142 = global read "_RT Global.vi" "ErrorMsg"() -> (w88:string)
            n143 = Equal?(x=_RT_Instrument_State."Turbopump Ready-Waiting", y=w92) -> (x = y?=w91:bool)
            n144 = Equal?(x=_RT_Instrument_State."Roughing Pump Ready", y=w92) -> (x = y?=w90:bool)
            n145 = Or(x=w91, y=w90) -> (x .or. y?=w89:bool)
            n146 = Equal?(x=_RT_Instrument_State."24V Standby", y=w92) -> (x = y?=w95:bool)
            n147 = Equal?(x=_RT_Instrument_State."Turbopump Ready", y=w92) -> (x = y?=w103:bool)
            n148 = Equal?(x=_RT_Instrument_State."Source Standby", y=w92) -> (x = y?=w102:bool)
            n149 = Select(t=w88, s=w89, f="") -> (s? t:f=w86:string)
            n150 = Or(x=w103, y=w102) -> (x .or. y?=w101:bool)
            n151 = Select(t=_RT_Instrument_State."Starting Up" ("x"), s=w95, f=w92) -> (s? t:f=w96:T3)
            n152 = Select(t=_RT_Instrument_State."Checking Vacuum" ("x"), s=w101, f=w96) -> (s? t:f=w99:T3)
          }
          frame 10 {
            w110 = FALSE
            # "Fatal Error"
            n153 = call "_FPGA Turbo Control.vi"("Command"=_Pump_Parameter."Turn Pump Motor Off") -> ("error out"=w107:errorcluster)  [unwired: 3 in, 5 out]
            n154 = call "_FPGA Set Parameters.vi"("ExhaustGas (on)"=w110, "CurGas (on)"=w110, "error in"=w107, "HSID Temp (on)"=w110) -> ("error out"=w106:errorcluster)  [unwired: 5 in, 2 out]
            n155 = call "_FPGA Toggle Electronics.vi"("error in"=w106) -> ()  [unwired: 2 in, 6 out]
          }
          frame 20 {
            n156 = call "_FPGA Turbo Control.vi"("Command"=_Pump_Parameter."Turn Pump Motor Off") -> ("error out"=w112:errorcluster)  [unwired: 3 in, 5 out]
            n157 = call "_FPGA Set LEDs.vi"("error in (no error)"=w112, "LED Command"=_LED_States."Solid R") -> ()  [unwired: 2 in, 4 out]
          }
          frame 32 {
            w122 = _RT_Instrument_State."24V Standby" ("x")
            w126 = FALSE ("ExhaustGas (on)")
            n158 = global read "_RT Global.vi" "StartupMode"() -> (w119:u8)
            n159 = call "_FPGA Set LEDs.vi"("LED Command"=_LED_States."Solid R") -> ("error out"=w127:errorcluster)  [unwired: 3 in, 3 out]
            n160 = Equal?(x=w122, y=w124) -> (x = y?=w123:bool)
            n161 = Select(t=w122, s=w123, f=w121) -> (s? t:f=w120:T3)
            n162 = call "_FPGA Set Parameters.vi"("ExhaustGas (on)"=w126, "CurGas (on)"=w126, "error in"=w127, "HSID Temp (on)"=w126) -> ()  [unwired: 5 in, 3 out]
            n163 = Max & Min(x=w119, y=u8 1 ("StartupMode")) -> (max(x,y)=w117:u8)  [unwired: 1 out]
            n164 = global write "_RT Global.vi" "StartupMode"(w117) -> ()
          }
          frame 35, 39 {
            n165 = global read "_RT Global.vi" "StartupMode"() -> (w131:u8)
            n166 = call "_FPGA Check Source ID.vi"() -> ("Source ID OK"=w134:bool)  [unwired: 1 in]
            n167 = call "_FPGA Set LEDs.vi"("LED Command"=_LED_States."Solid R") -> ("error out"=w136:errorcluster)  [unwired: 3 in, 3 out]
            n168 = call "_FPGA Set Parameters.vi"("ExhaustGas (on)"=FALSE, "error in"=w136, "HSID Temp (on)"=w134) -> ()  [unwired: 6 in, 3 out]
            n169 = Max & Min(x=w131, y=u8 1 ("StartupMode")) -> (max(x,y)=w129:u8)  [unwired: 1 out]
            n170 = global write "_RT Global.vi" "StartupMode"(w129) -> ()
          }
          frame 40 {
            # "Going to source standby state"
            n171 = global read "_RT Global.vi" "StartupMode"() -> (w141:u8)
            n172 = call "_FPGA Set Parameters.vi"("Source Standby (F)"=TRUE, "HSID Temp (on)"=FALSE) -> ("error out"=w138:errorcluster)  [unwired: 7 in, 2 out]
            n173 = Max & Min(x=w141, y=u8 1 ("StartupMode")) -> (max(x,y)=w139:u8)  [unwired: 1 out]
            n174 = global write "_RT Global.vi" "StartupMode"(w139) -> ()
            n175 = call "_FPGA Set LEDs.vi"("error in (no error)"=w138, "LED Command"=_LED_States."Solid R") -> ()  [unwired: 2 in, 4 out]
          }
        }
        n176 = global write "_RT Global.vi" "ErrorMsg"(w53) -> ()
      }
    }
  }
  "Next InstrState" <- w1
  "Running" <- w5
  n177 = local read "CurInstrState"() -> (w3:T3)
  n178 = Not Equal?(x=w1, y=w3) -> (x != y?=w2:bool)
  n179 = case shown="True" w2 {
    tunnel: w1 -> [_ w348]
    frame False {
    }
    frame True {
      n180 = case shown="\"Lost Communication\"" w348 {
        frame "Initializing", Default {
        }
        frame "Turbopump Ready" {
          n181 = call "_RT Event.vi"("Event"="Going to Turbopump Ready state.") -> ()  [unwired: 2 in, 5 out]
        }
        frame "Lost Communication" {
          n182 = call "_RT Event.vi"("Event"="Going to Lost Communication state.") -> ()  [unwired: 2 in, 5 out]
        }
        frame "Turbopump Ready-Waiting" {
          n183 = call "_RT Event.vi"("Event"="Going to Turbopump Ready-Waiting state.") -> ()  [unwired: 2 in, 5 out]
        }
        frame "Source Standby" {
          n184 = call "_RT Event.vi"("Event"="Going to Source Standby state.") -> ()  [unwired: 2 in, 5 out]
        }
      }
    }
  }
